vi "HandleItemActivation.vi"(8 "error in (no error)":errorcluster, 11 "RingItemProjectWizard in":refnum<class "RingItemProjectWizard.lvclass">) -> (0 "error out":errorcluster, 3 "RingItemProjectWizard out":refnum<class "RingItemProjectWizard.lvclass">)   [LabVIEW 2009, in "NavScreen.lvlib" / "RingItemProjectWizard.lvclass"]
uses:
  RingItemProjectWizard.lvclass
  RingItemProjectWizard.lvclass/RingItemProjectWizard.ctl
  ProjectWizard/ProjectWizard.lvclass
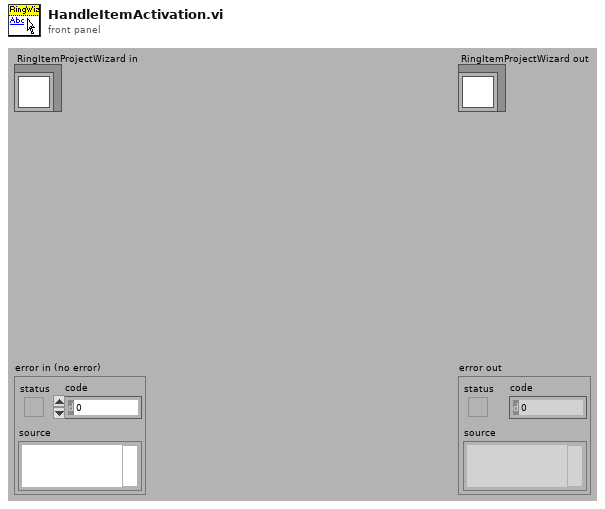
[diagram p1: front panel]
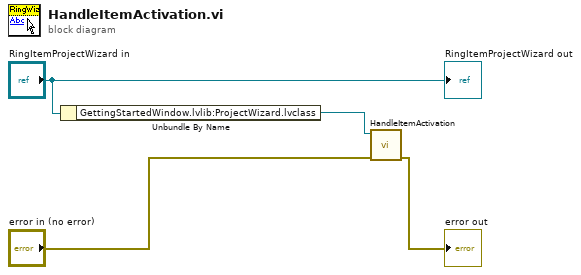
[diagram p0: block diagram]
diagram:
  n1 = Unbundle By Name("RingItemProjectWizard in") -> ("GettingStartedWindow.lvlib:ProjectWizard.lvclass"=w4:refnum<class "ProjectWizard.lvclass">)
  n2 = call "HandleItemActivation.vi"("error in (no error)"="error in (no error)", "GettingStartedWindow.lvlib:ProjectWizard.lvclass"=w4) -> ("error out"=→"error out":errorcluster)  [unwired: 8 in, 1 out]
  "RingItemProjectWizard out" <- "RingItemProjectWizard in"
